vi "Stop TDSM.vi"(8 "error in":errorcluster, 11 "UDP Reader in":refnum<class "UDP Reader.lvclass">) -> (0 "error out":errorcluster, 3 "UDP Reader out":refnum<class "UDP Reader.lvclass">)   [LabVIEW 2022 SP3, in "UDP Reader.lvlib" / "UDP Reader.lvclass"]
uses:
  UDP Reader.lvclass
  C:/Program Files (x86)/National Instruments/LabVIEW 2022/vi.lib/ActorFramework/Actor/Actor.lvclass
  <vilib>/ActorFramework/Actor/Actor.lvclass/Actor.ctl
  UDP Reader.lvclass/UDP Reader.ctl
  UDP Data Receiver/UDP Data Receiver Messages/RX Msg/RX Msg.lvclass/RX Msg.ctl
  <vilib>/ActorFramework/Message Enqueuer/Message Enqueuer.lvclass/Message Enqueuer.ctl
  <vilib>/ActorFramework/Time-Delayed Send Message/Time-Delay Override Options.ctl
  <vilib>/ActorFramework/Message Enqueuer/Enqueue.vi
  UDP Data Receiver/UDP Data Receiver Messages/RX Msg/RX Msg.lvclass
  C:/Program Files (x86)/National Instruments/LabVIEW 2022/vi.lib/ActorFramework/Message/Message.lvclass
  <vilib>/ActorFramework/Message Priority Queue/Priority Enqueue.vi
  <vilib>/ActorFramework/Actor/Actor.lvclass
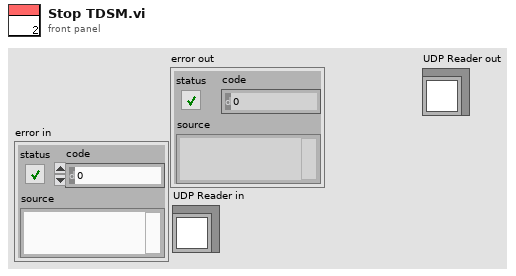
[diagram p1: front panel]
types:
  T1 = typedef "Time-Delay Override Options.ctl" = enum16{"Send next copy now", "Skip next scheduled copy", "Send next copy now and stop all further copies", "Stop all further copies"}
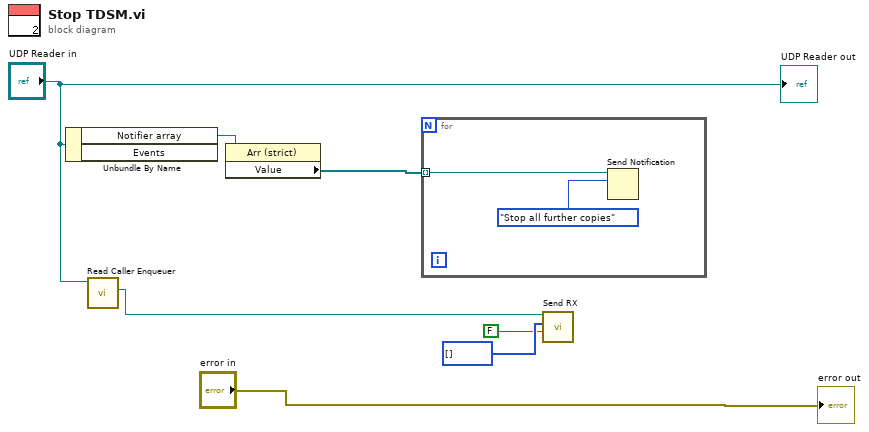
[diagram p0: block diagram]
diagram:
  n1 = Unbundle By Name("UDP Reader in") -> ("Notifier array"=w7:refnum<vi>)  [unwired: 1 out]
  n2 = call <vilib>:"Read Caller Enqueuer.vi"("Actor"="UDP Reader in") -> ("Caller Enqueuer"=w3:refnum<class "Message Enqueuer.lvclass">)  [unwired: 10 in]
  n3 = property class="Arr (strict)"(reference=w7) -> ("Value"=w5:refnum<notifier>[])  [unwired: 1 in, 2 out]
  n4 = for {
    tunnel: w5 -> [w8] mode=indexing
    n5 = Send Notification(notification=Time-Delay_Override_Options."Stop all further copies", notifier=w8) -> ()  [unwired: 1 in, 2 out]
  }
  n6 = call "Send RX.vi"("RX"=FALSE, "Data"=u8[] [], "Message Enqueuer"=w3) -> ()  [unwired: 7 in, 2 out]
  "UDP Reader out" <- "UDP Reader in"
  "error out" <- "error in"
